vi "Trigger_Loggic.vi"(8 "error in (no error)":errorcluster) -> (0 "error out":errorcluster, 3 "Array":i32[](array[numeric]))   [LabVIEW 2017]
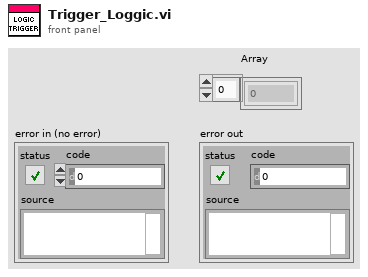
[diagram p1: front panel]
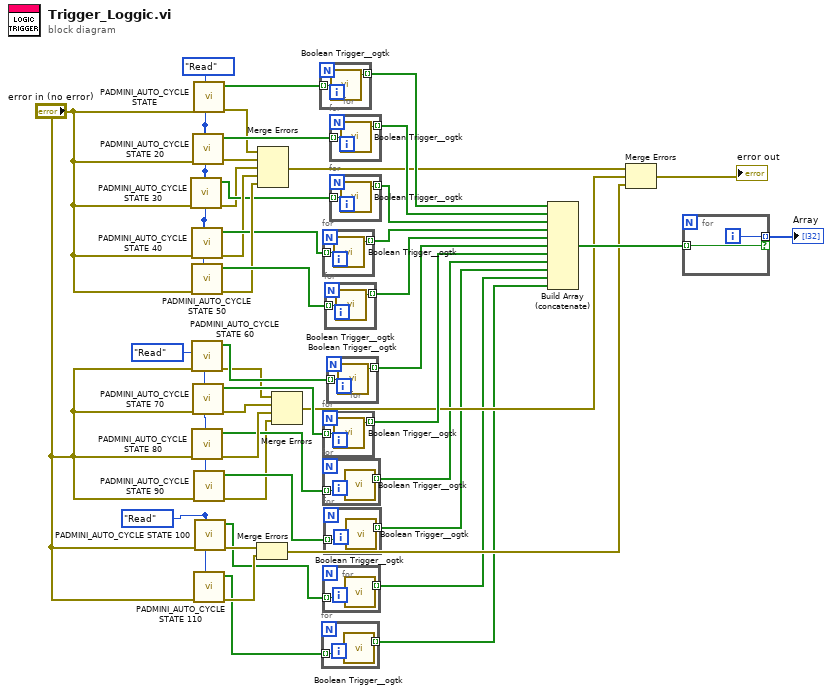
[diagram p0: block diagram]
diagram:
  w1 = enum16{"Read", "Write"}."Read" ("Enum")
  w2 = enum16{"Read", "Write"}."Read" ("Enum")
  w5 = enum16{"Read", "Write"}."Read" ("Enum")
  n1 = call "PADMINI_AUTO_CYCLE STATE 30.vi"("Enum"=w5, "error in (no error)"="error in (no error)") -> ("error out"=w31:errorcluster, "Input 2"=w32:bool[])  [unwired: 8 in]
  n2 = call "PADMINI_AUTO_CYCLE STATE 40.vi"("Enum"=w5, "error in (no error)"="error in (no error)") -> ("error out"=w34:errorcluster, "Input 2"=w35:bool[])  [unwired: 8 in]
  n3 = call "PADMINI_AUTO_CYCLE STATE 50.vi"("Enum"=w5, "error in (no error)"="error in (no error)") -> ("error out"=w37:errorcluster, "Input 2"=w38:bool[])  [unwired: 8 in]
  n4 = call "PADMINI_AUTO_CYCLE STATE 60.vi"("Enum"=w2, "error in (no error)"="error in (no error)") -> ("error out"=w22:errorcluster, "Input 2"=w40:bool[])  [unwired: 8 in]
  n5 = call "PADMINI_AUTO_CYCLE STATE 80.vi"("Enum"=w2, "error in (no error)"="error in (no error)") -> ("error out"=w17:errorcluster, "Input 2"=w16:bool[])  [unwired: 8 in]
  n6 = call "PADMINI_AUTO_CYCLE STATE 20.vi"("Enum"=w5, "error in (no error)"="error in (no error)") -> ("error out"=w25:errorcluster, "Input 2"=w27:bool[])  [unwired: 8 in]
  n7 = call "PADMINI_AUTO_CYCLE STATE 70.vi"("Enum"=w2, "error in (no error)"="error in (no error)") -> ("error out"=w21:errorcluster, "Input 2"=w42:bool[])  [unwired: 8 in]
  n8 = call "PADMINI_AUTO_CYCLE STATE.vi"("Enum"=w5, "error in (no error)"="error in (no error)") -> ("error out"=w26:errorcluster, "Input 2"=w29:bool[])  [unwired: 8 in]
  n9 = call "PADMINI_AUTO_CYCLE STATE 90.vi"("Enum"=w2, "error in (no error)"="error in (no error)") -> ("error out"=w11:errorcluster, "Input 2"=w14:bool[])  [unwired: 8 in]
  n10 = call "PADMINI_AUTO_CYCLE STATE 110.vi"("Enum"=w1, "error in (no error)"="error in (no error)") -> ("error out"=w10:errorcluster, "Input 2"=w6:bool[])  [unwired: 8 in]
  n11 = call "PADMINI_AUTO_CYCLE STATE 100.vi"("Enum"=w1, "error in (no error)"="error in (no error)") -> ("error out"=w9:errorcluster, "Input 2"=w7:bool[])  [unwired: 8 in]
  n12 = Merge Errors(w9, w10) -> (w8:errorcluster)
  n13 = Merge Errors(w26, w25, w31, w34, w37) -> (w19:errorcluster)
  n14 = Merge Errors(w22, w21, w17, w11) -> (w20:errorcluster)
  n15 = for {
    tunnel: w29 -> [w45] mode=indexing
    tunnel: [w44] -> w30 mode=indexing
    n16 = call <userlib>:"Boolean Trigger__ogtk.vi"("Boolean Input"=w45) -> ("Rising Edge"=w44:bool)  [unwired: 1 in, 1 out]
  }
  n17 = for {
    tunnel: w6 -> [w47] mode=indexing
    tunnel: [w46] -> w3 mode=indexing
    n18 = call <userlib>:"Boolean Trigger__ogtk.vi"("Boolean Input"=w47) -> ("Rising Edge"=w46:bool)  [unwired: 1 in, 1 out]
  }
  n19 = for {
    tunnel: w35 -> [w49] mode=indexing
    tunnel: [w48] -> w36 mode=indexing
    n20 = call <userlib>:"Boolean Trigger__ogtk.vi"("Boolean Input"=w49) -> ("Rising Edge"=w48:bool)  [unwired: 1 in, 1 out]
  }
  n21 = for {
    tunnel: w42 -> [w51] mode=indexing
    tunnel: [w50] -> w43 mode=indexing
    n22 = call <userlib>:"Boolean Trigger__ogtk.vi"("Boolean Input"=w51) -> ("Rising Edge"=w50:bool)  [unwired: 1 in, 1 out]
  }
  n23 = for {
    tunnel: w16 -> [w53] mode=indexing
    tunnel: [w52] -> w15 mode=indexing
    n24 = call <userlib>:"Boolean Trigger__ogtk.vi"("Boolean Input"=w53) -> ("Rising Edge"=w52:bool)  [unwired: 1 in, 1 out]
  }
  n25 = for {
    tunnel: w7 -> [w55] mode=indexing
    tunnel: [w54] -> w4 mode=indexing
    n26 = call <userlib>:"Boolean Trigger__ogtk.vi"("Boolean Input"=w55) -> ("Rising Edge"=w54:bool)  [unwired: 1 in, 1 out]
  }
  n27 = for {
    tunnel: w14 -> [w57] mode=indexing
    tunnel: [w56] -> w13 mode=indexing
    n28 = call <userlib>:"Boolean Trigger__ogtk.vi"("Boolean Input"=w57) -> ("Rising Edge"=w56:bool)  [unwired: 1 in, 1 out]
  }
  n29 = for {
    tunnel: w38 -> [w59] mode=indexing
    tunnel: [w58] -> w39 mode=indexing
    n30 = call <userlib>:"Boolean Trigger__ogtk.vi"("Boolean Input"=w59) -> ("Rising Edge"=w58:bool)  [unwired: 1 in, 1 out]
  }
  n31 = for {
    tunnel: w40 -> [w61] mode=indexing
    tunnel: [w60] -> w41 mode=indexing
    n32 = call <userlib>:"Boolean Trigger__ogtk.vi"("Boolean Input"=w61) -> ("Rising Edge"=w60:bool)  [unwired: 1 in, 1 out]
  }
  n33 = for {
    tunnel: w27 -> [w63] mode=indexing
    tunnel: [w62] -> w28 mode=indexing
    n34 = call <userlib>:"Boolean Trigger__ogtk.vi"("Boolean Input"=w63) -> ("Rising Edge"=w62:bool)  [unwired: 1 in, 1 out]
  }
  n35 = for {
    tunnel: w32 -> [w65] mode=indexing
    tunnel: [w64] -> w33 mode=indexing
    n36 = call <userlib>:"Boolean Trigger__ogtk.vi"("Boolean Input"=w65) -> ("Rising Edge"=w64:bool)  [unwired: 1 in, 1 out]
  }
  n37 = Build Array (concatenate)(w30, w28, w33, w36, w39, w41, w43, w15, w13, w4, w3) -> (w24:bool[])
  n38 = Merge Errors(w19, w20, w8) -> (→"error out":errorcluster)
  n39 = for {
    tunnel: w24 -> [w66] mode=indexing
    tunnel: [w67] -> w23 mode=indexing if=w66
    i -> [w67]
  }
  "Array" <- w23
